vi "Read Room Number.vi"(8 "error in (no error)":errorcluster, 11 "Flags in":refnum<class "Flags.lvclass">) -> (0 "error out":errorcluster, 2 "Room Number":u32, 3 "Flags out":refnum<class "Flags.lvclass">)   [LabVIEW 2015]
uses:
  Flags.lvclass
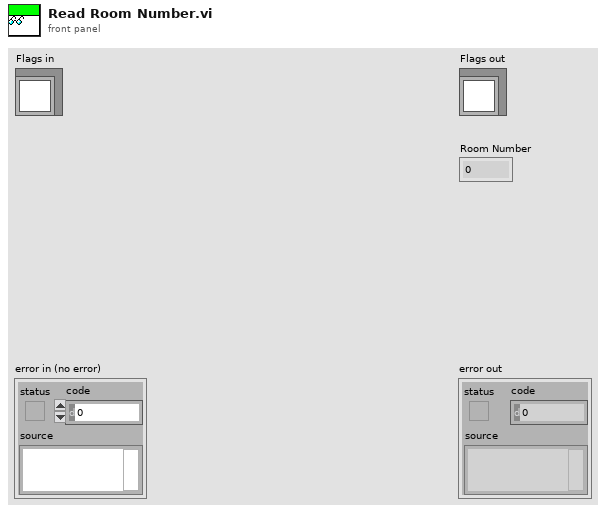
[diagram p1: front panel]
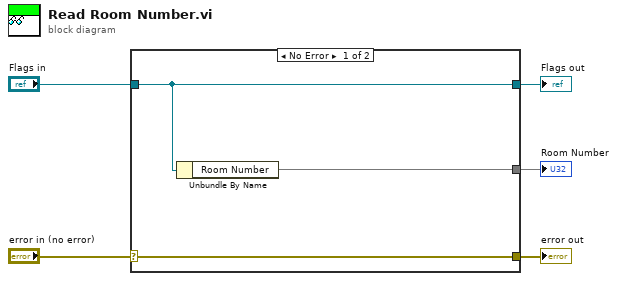
[diagram p0: block diagram]
diagram:
  n1 = case shown="No Error" "error in (no error)" {
    selector: "error in (no error)" -> [w8 w9]
    tunnel: [w8 w9] -> w4
    tunnel: [w7 w10] -> w2
    tunnel: "Flags in" -> [w7 w10]
    tunnel: [w6 _] -> w1
    frame No Error {
      n2 = Unbundle By Name(w7) -> ("Room Number"=w6)
    }
    frame Error {
    }
  }
  "error out" <- w4
  "Flags out" <- w2
  "Room Number" <- w1
